vi "EE_DataDisplayingLoop.vi"(0 "ChannelsDataNotifier in":T1, 5 "EEG Waveform Chart Refnum":refnum<vi>, 9 "Wireless Signal Strength":refnum<vi>, 11 "StopButton Refnum":refnum<vi>, 12 "Error Message Refnum":refnum<vi>) -> (4 "ChannelsDataNotifier out":T1, 15 "error out":errorcluster)   [LabVIEW 2016, in "Emotiv Epoc.lvlib"]
uses:
  EE_Notifier_Refnum.ctl
  EE_Notifier_Data_Type.ctl
  EE_SignalStrength_enum.ctl
  EE_EEG_ContactQuality_enum.ctl
  Emotiv Epoc.lvlib
  EmotivEpocHeadsetControls.lvclass
panel:
  # "This VI is a part of BCI Design library, http://www.ru-bci.org \nCopyright © 2020, Sotnikov Peter, All rights reserved. License: CC BY-NC 4.0"
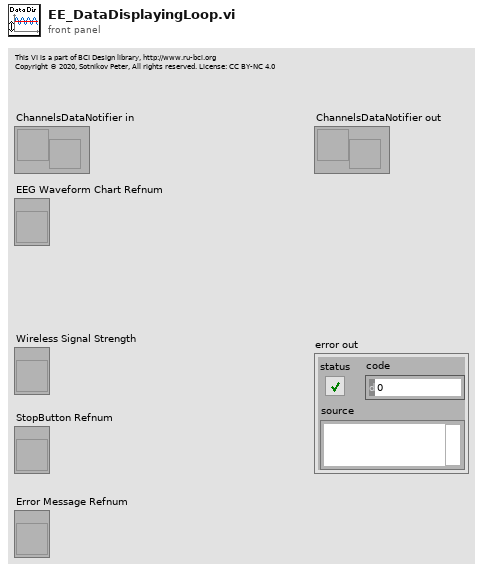
[diagram p1: front panel]
types:
  T1 = typedef "Emotiv Epoc.lvlib/EE_Notifier_Refnum.ctl" = refnum<notifier>
  T2 = typedef "Emotiv Epoc.lvlib/EE_Notifier_Data_Type.ctl" = cluster{"EDK_Error":string, "Number of samples":u32, "Marker Waveform":waveform(dbl), "Array of EEG waveforms":waveform(dbl)[], "WirelessSignalStatus":T3, "EEG_ContactsQuality":T4[]}
  T3 = typedef "Emotiv Epoc.lvlib/EmotivEpocHeadsetControls.lvclass/EE_SignalStrength_enum.ctl" = enum32{"NO_SIGNAL", "BAD_SIGNAL", "GOOD_SIGNAL"}
  T4 = typedef "Emotiv Epoc.lvlib/EE_EEG_ContactQuality_enum.ctl" = enum16{"EEG_CQ_NO_SIGNAL", "EEG_CQ_VERY_BAD", "EEG_CQ_POOR", "EEG_CQ_FAIR", "EEG_CQ_GOOD"}
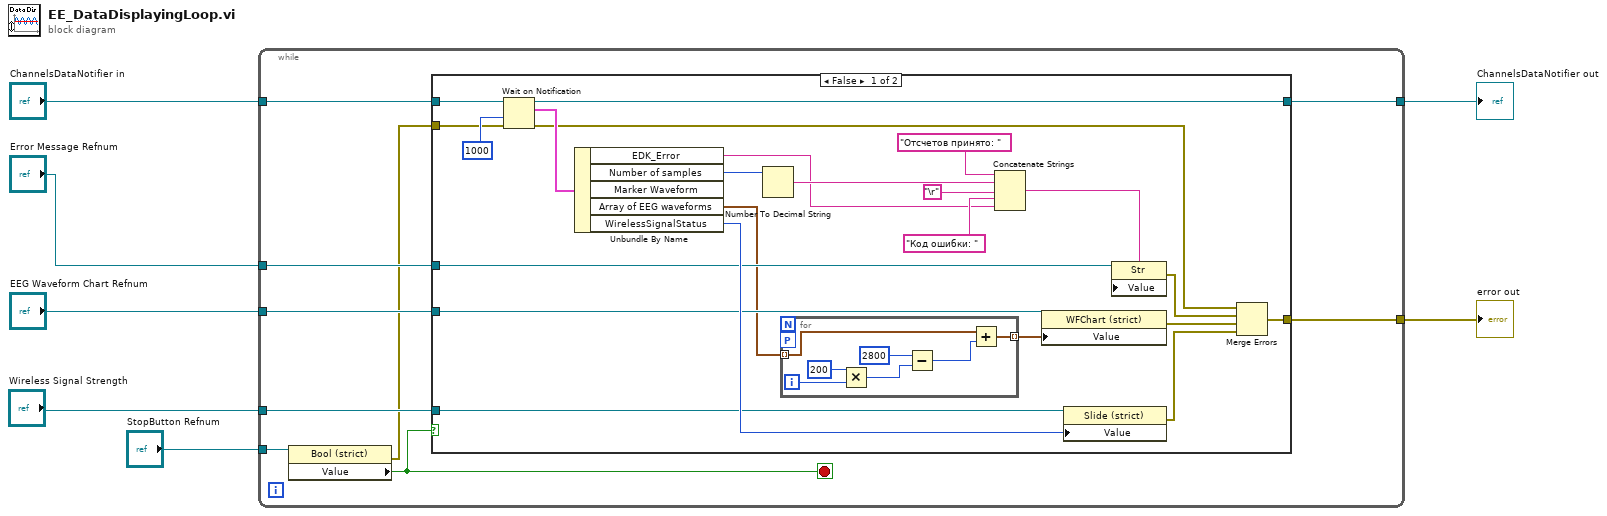
[diagram p0: block diagram]
diagram:
  n1 = while {
    tunnel: "StopButton Refnum" -> [w16]
    tunnel: [w8] -> w6
    tunnel: "ChannelsDataNotifier in" -> [w15]
    tunnel: [w14] -> w4
    tunnel: "Wireless Signal Strength" -> [w13]
    tunnel: "Error Message Refnum" -> [w12]
    tunnel: "EEG Waveform Chart Refnum" -> [w11]
    stop <- w10 stop-if-true
    n2 = property class="Bool (strict)"(reference=w16) -> (error out=w9:errorcluster, "Value"=w10:bool)  [unwired: 1 in, 1 out]
    n3 = case shown="False" w10 {
      tunnel: w15 -> [w39 w48]
      tunnel: [w37 w48] -> w14
      tunnel: w13 -> [w34 _]
      tunnel: w12 -> [w31 _]
      tunnel: w11 -> [w30 _]
      tunnel: w9 -> [w22 w47]
      tunnel: [w18 w47] -> w8
      frame False {
        n4 = Wait on Notification(notifier=w39, timeout in ms (-1)=1000, error in (no error)=w22) -> (notifier out=w37:T1, notification=w36:T2, error out=w17:errorcluster)  [unwired: 1 in, 1 out]
        n5 = Unbundle By Name(w36) -> ("EDK_Error"=w23:string, "Number of samples"=w33:u32, "Array of EEG waveforms"=w28:waveform(dbl)[], "WirelessSignalStatus"=w35:T3)  [unwired: 1 out]
        n6 = Number To Decimal String(number=w33) -> (decimal integer string=w26:string)  [unwired: 1 in]
        n7 = for {
          tunnel: [w42] -> w29 mode=indexing
          tunnel: w28 -> [w41] mode=indexing
          workers-P: _ -> [_]
          i -> [w46]
          n8 = Multiply(x=200, y=w46) -> (x*y=w44:i32)
          n9 = Subtract(x=2800, y=w44) -> (x-y=w40:i32)
          n10 = Add(x=w41, y=w40) -> (x+y=w42:waveform(dbl))
        }
        n11 = Concatenate Strings("Отсчетов принято: " ("string"), w26, "\r", "Код ошибки: " ("string"), w23) -> (w32:string)
        n12 = property class="WFChart (strict)"(reference=w30, "Value"=w29) -> (error out=w20:errorcluster)  [unwired: 1 in, 1 out]
        n13 = property class="Slide (strict)"(reference=w34, "Value"=w35) -> (error out=w21:errorcluster)  [unwired: 1 in, 1 out]
        n14 = property class="Str"(reference=w31, "Value"=w32) -> (error out=w19:errorcluster)  [unwired: 1 in, 1 out]
        n15 = Merge Errors(w17, w19, w20, w21) -> (w18:errorcluster)
      }
      frame True {
      }
    }
  }
  "error out" <- w6
  "ChannelsDataNotifier out" <- w4
